vi "query.vi"(8 "error in (no error)":errorcluster, 10 "SQL Statement":string, 11 "object in":refnum<class "SQLiteConnection.lvclass">) -> (0 "error out":errorcluster, 1 "names":string[](array[string]), 2 "result":string[][](array[string]), 3 "object out":refnum<class "SQLiteConnection.lvclass">)   [LabVIEW 2019, in "SQLiteConnection.lvclass"]
uses:
  SQLiteConnection.lvclass
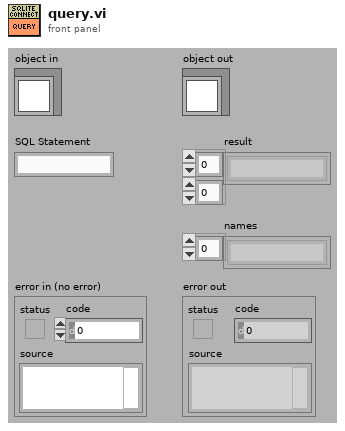
[diagram p1: front panel]
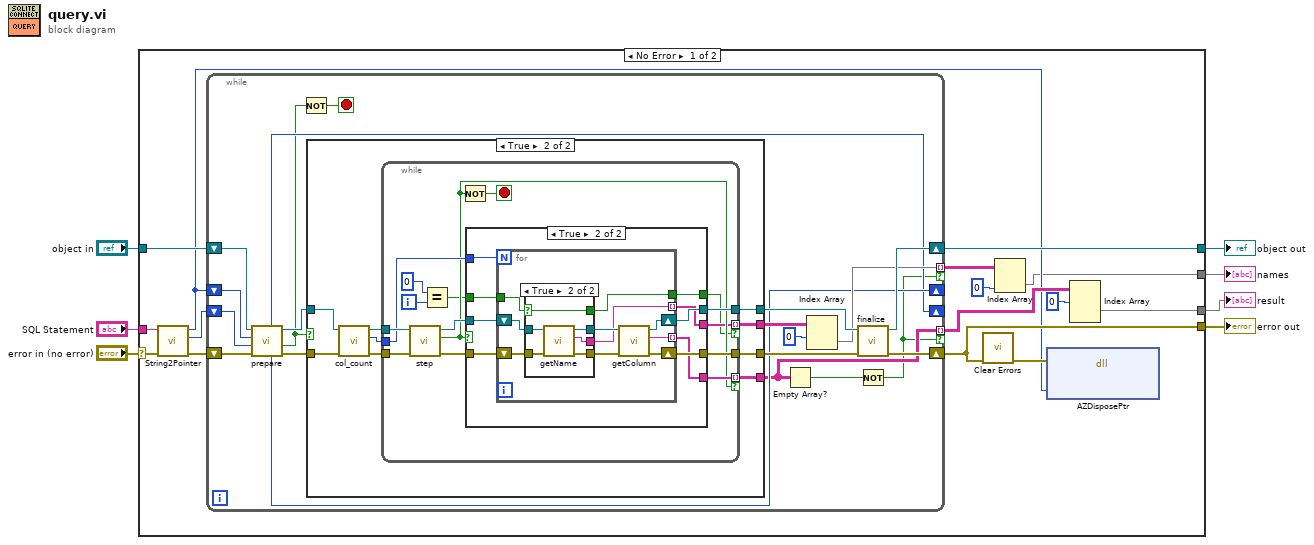
[diagram p0: block diagram]
diagram:
  n1 = case shown="No Error" "error in (no error)" {
    selector: "error in (no error)" -> [w16 w100]
    tunnel: [w18 w100] -> w6
    tunnel: [w20 w99] -> w4
    tunnel: "object in" -> [w21 w99]
    tunnel: "SQL Statement" -> [w14 _]
    tunnel: [w11 _] -> w2
    tunnel: [w9 _] -> w1
    frame No Error {
      n2 = call "String2Pointer.vi"("error in (no error)"=w16, "SQL Statement"=w14) -> ("error out"=w15:errorcluster, "size"=w13:i32, "pointer"=w12:i64)  [unwired: 7 in]
      n3 = while {
        tunnel: [w25] -> w22 mode=indexing if=w23
        tunnel: [w32] -> w19 mode=indexing if=w23
        shift-right: [w31] -> w18
        shift-left: w15 -> [w37]
        shift-right: [w35] -> w20
        shift-left: w21 -> [w36]
        shift-right: [w28] -> _
        shift-left: w12 -> [w42]
        shift-right: [w27] -> _
        shift-left: w13 -> [w29]
        stop <- w30 stop-if-true
        n4 = call "prepare.vi"("error in (no error)"=w37, "length"=w29, "sqlstatement pointer"=w42, "object in"=w36) -> ("error out"=w41:errorcluster, "Valid?"=w26:bool, "object out"=w40:refnum<class "SQLiteConnection.lvclass">, "remaining sql"=w28:i64, "remaining bytes"=w27:i32)  [unwired: 3 in]
        n5 = Not(x=w26) -> (.not. x?=w30:bool)
        n6 = case shown="True" w26 {
          tunnel: w41 -> [w44 w53]
          tunnel: w40 -> [w43 w52]
          tunnel: [w44 w48] -> w39
          tunnel: [w43 w47] -> w38
          tunnel: [_ w46] -> w25
          tunnel: [_ w45] -> w34
          frame False {
          }
          frame True {
            n7 = call "col_count.vi"("error in (no error)"=w53, "object in"=w52) -> ("error out"=w50:errorcluster, "column count"=w49:i32, "object out"=w51:refnum<class "SQLiteConnection.lvclass">)  [unwired: 7 in]
            n8 = while {
              tunnel: w50 -> [w68]
              tunnel: w51 -> [w67]
              tunnel: w49 -> [w65]
              tunnel: [w62] -> w47
              tunnel: [w61] -> w48
              tunnel: [w60] -> w46 mode=indexing if=w59
              tunnel: [w55] -> w45 mode=indexing if=w54
              i -> [w58]
              stop <- w66 stop-if-true
              n9 = call "step.vi"("error in (no error)"=w68, "object in"=w67) -> ("error out"=w64:errorcluster, "row?"=w59:bool, "object out"=w63:refnum<class "SQLiteConnection.lvclass">)  [unwired: 7 in]
              n10 = Equal?(x=0, y=w58) -> (x = y?=w56:bool)
              n11 = Not(x=w59) -> (.not. x?=w66:bool)
              n12 = case shown="True" w59 {
                tunnel: w65 -> [_ w79]
                tunnel: w64 -> [w69 w78]
                tunnel: w63 -> [w70 w77]
                tunnel: [w70 w76] -> w62
                tunnel: [w69 w75] -> w61
                tunnel: [_ w74] -> w60
                tunnel: w56 -> [_ w73]
                tunnel: [_ w72] -> w55
                tunnel: [_ w71] -> w54
                frame False {
                }
                frame True {
                  n13 = for {
                    N: w79 -> [_]
                    shift-right: [w88] -> w76
                    shift-left: w77 -> [w83]
                    shift-right: [w89] -> w75
                    shift-left: w78 -> [w85]
                    tunnel: [w87] -> w74 mode=indexing
                    tunnel: w73 -> [w86]
                    tunnel: [w81] -> w72 mode=indexing
                    tunnel: [w80] -> w71
                    n14 = case shown="True" w86 {
                      selector: w86 -> [w90 w94]
                      tunnel: w85 -> [w91 w98]
                      tunnel: [w91 w97] -> w84
                      tunnel: w83 -> [w92 w96]
                      tunnel: [w92 w95] -> w82
                      tunnel: [w90 w94] -> w80
                      tunnel: [_ w93] -> w81
                      frame False {
                      }
                      frame True {
                        n15 = call "getName.vi"("error in (no error)"=w98, "object in"=w96) -> ("error out"=w97:errorcluster, "col name"=w93:string, "object out"=w95:refnum<class "SQLiteConnection.lvclass">)  [unwired: 7 in]
                      }
                    }
                    n16 = call "getColumn.vi"("error in (no error)"=w84, "object in"=w82) -> ("error out"=w89:errorcluster, "col text"=w87:string, "object out"=w88:refnum<class "SQLiteConnection.lvclass">)  [unwired: 7 in]
                  }
                }
              }
            }
          }
        }
        n17 = Empty Array?(array=w25) -> (empty?=w24:bool)
        n18 = Index Array(array=w34, index (row)=0) -> (element=w32:string[])  [unwired: 1 in]
        n19 = call-dynamic "finalize.vi"("error in (no error)"=w39, "object in"=w38) -> ("error out"=w31:errorcluster, "object out"=w35:refnum<class "SQLiteConnection.lvclass">)  [unwired: 8 in]
        n20 = Not(x=w24) -> (.not. x?=w23:bool)
      }
      n21 = call <vilib>:"Clear Errors.vi"("error in (no error)"=w18) -> ("error out"=w17:errorcluster)  [unwired: 5 in, 1 out]
      n22 = Index Array(array=w19, index (col)=0 ("disabled index (col)")) -> (element=w9:string[])  [unwired: 1 in]
      n23 = dll-call lib="LabVIEW" fn="AZDisposePtr"(error in=w17, "pointer"=w12) -> ()  [unwired: 4 in, 2 out]
      n24 = Index Array(array=w22, index (dim 0)=0 ("index (page)")) -> (element=w11:string[][])  [unwired: 2 in]
    }
    frame Error {
    }
  }
  "error out" <- w6
  "object out" <- w4
  "result" <- w2
  "names" <- w1
